vi "Generate random pts inside tri.vi"(1 "V2":sgl[](array[numeric]), 2 "V1":sgl[](array[numeric]), 3 "V0":sgl[](array[numeric]), 4 "N pts":i32) -> (0 "Pts":sgl[][](array[numeric]))   [LabVIEW 2017]
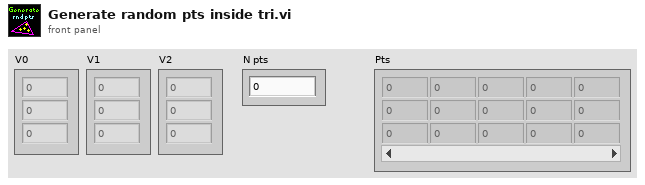
[diagram p1: front panel]
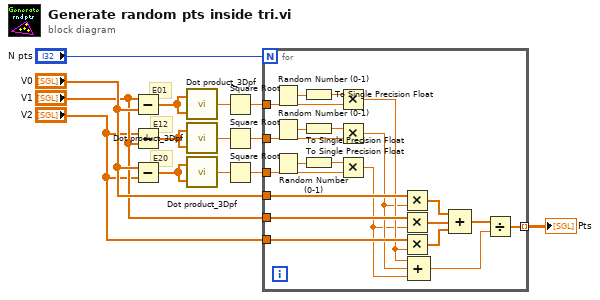
[diagram p0: block diagram]
diagram:
  # "E20"
  # "E12"
  # "E01"
  n1 = Subtract(x="V1", y="V0") -> (x-y=w10:sgl[])
  n2 = Subtract(x="V2", y="V1") -> (x-y=w9:sgl[])
  n3 = Subtract(x="V0", y="V2") -> (x-y=w8:sgl[])
  n4 = call "Dot product_3Dpf.vi"("B"=w10, "A"=w10) -> ("A . B"=w7:sgl)
  n5 = call "Dot product_3Dpf.vi"("B"=w9, "A"=w9) -> ("A . B"=w6:sgl)
  n6 = call "Dot product_3Dpf.vi"("B"=w8, "A"=w8) -> ("A . B"=w5:sgl)
  n7 = Square Root(x=w7) -> (sqrt(x)=w4:sgl)
  n8 = Square Root(x=w6) -> (sqrt(x)=w3:sgl)
  n9 = Square Root(x=w5) -> (sqrt(x)=w2:sgl)
  n10 = for {
    N: "N pts" -> [_]
    tunnel: "V0" -> [w35]
    tunnel: "V1" -> [w34]
    tunnel: "V2" -> [w33]
    tunnel: [w32] -> w11 mode=indexing
    tunnel: w4 -> [w25]
    tunnel: w3 -> [w22]
    tunnel: w2 -> [w19]
    n11 = Random Number (0-1)() -> (number: 0 to 1=w26:dbl)
    n12 = Random Number (0-1)() -> (number: 0 to 1=w23:dbl)
    n13 = Random Number (0-1)() -> (number: 0 to 1=w20:dbl)
    n14 = To Single Precision Float(number=w26) -> (single precision float=w17:sgl)
    n15 = To Single Precision Float(number=w23) -> (single precision float=w16:sgl)
    n16 = To Single Precision Float(number=w20) -> (single precision float=w15:sgl)
    n17 = Multiply(x=w17, y=w25) -> (x*y=w24:sgl)
    n18 = Multiply(x=w16, y=w22) -> (x*y=w21:sgl)
    n19 = Multiply(x=w15, y=w19) -> (x*y=w18:sgl)
    n20 = Multiply(x=w35, y=w21) -> (x*y=w31:sgl[])
    n21 = Multiply(x=w34, y=w18) -> (x*y=w30:sgl[])
    n22 = Multiply(x=w33, y=w24) -> (x*y=w29:sgl[])
    n23 = Compound Arithmetic op=ADD(w24, w21, w18) -> (w27:sgl)
    n24 = Compound Arithmetic op=ADD(w31, w30, w29) -> (w28:sgl[])
    n25 = Divide(x=w28, y=w27) -> (x/y=w32:sgl[])
  }
  "Pts" <- w11
